vi "sub UI set title.vi"(8 "error in (no error)":errorcluster, 10 "title":T1, 11 "IDE simple in":refnum<class "LF2R IDE.lvclass">) -> (0 "error out":errorcluster, 3 "IDE simple out":refnum<class "LF2R IDE.lvclass">)   [LabVIEW 2018, in "LF2R IDE.lvlib" / "LF2R IDE.lvclass"]
uses:
  LF2R IDE.lvclass
  Frame Analizer/frame title.ctl
  LF2R IDE.lvclass/LF2R IDE.ctl
  Frame Analizer/Data Parser.lvclass
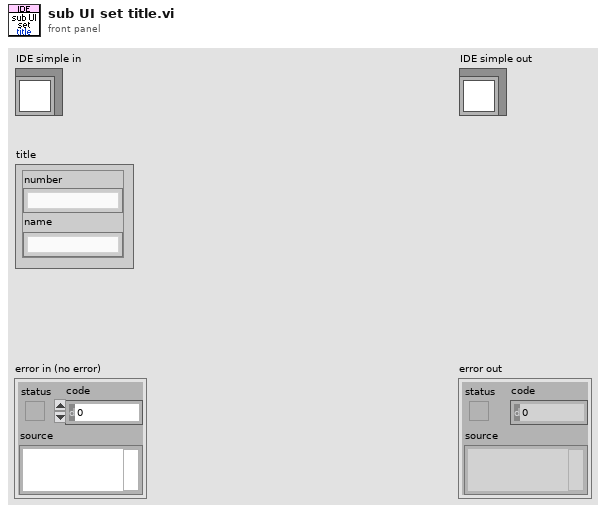
[diagram p1: front panel]
types:
  T1 = typedef "Data Parser.lvclass/frame title.ctl" = cluster{"number":string, "name":string}
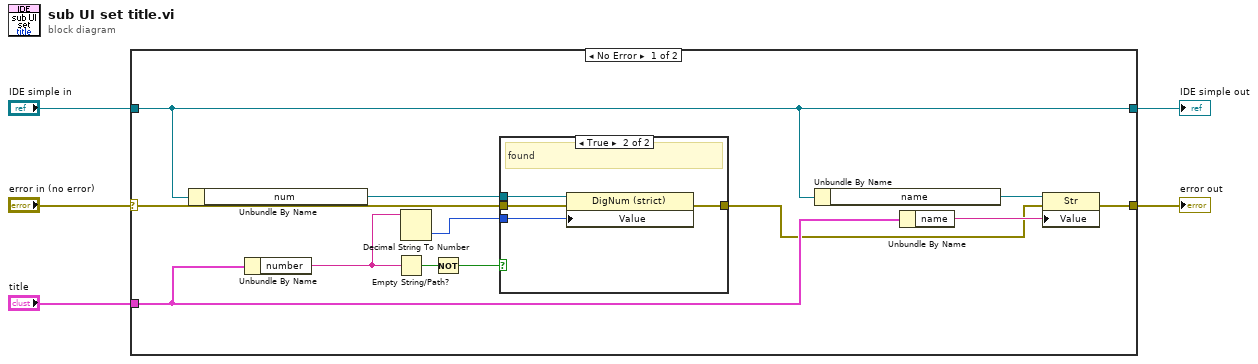
[diagram p0: block diagram]
diagram:
  n1 = case shown="No Error" "error in (no error)" {
    selector: "error in (no error)" -> [w7 w24]
    tunnel: [w15 w24] -> w4
    tunnel: [w14 w23] -> w2
    tunnel: "IDE simple in" -> [w14 w23]
    tunnel: "title" -> [w13 _]
    frame No Error {
      n2 = Unbundle By Name(w14) -> ("num"=w10:refnum<vi>)
      n3 = Unbundle By Name(w13) -> ("number"=w11:string)
      n4 = Empty String/Path?(string/path=w11) -> (empty?=w12:bool)
      n5 = Decimal String To Number(string=w11) -> (number=w8:i32)  [unwired: 2 in, 1 out]
      n6 = Not(x=w12) -> (.not. x?=w9:bool)
      n7 = case shown="True" w9 {
        tunnel: w10 -> [_ w22]
        tunnel: w8 -> [_ w21]
        tunnel: w7 -> [w18 w20]
        tunnel: [w18 w19] -> w6
        frame False {
          # "not found"
        }
        frame True {
          # "found"
          n8 = property class="DigNum (strict)"(reference=w22, error in=w20, "Value"=w21) -> (error out=w19:errorcluster)  [unwired: 1 out]
        }
      }
      n9 = Unbundle By Name(w14) -> ("name"=w17:refnum<vi>)
      n10 = Unbundle By Name(w13) -> ("name"=w16:string)
      n11 = property class="Str"(reference=w17, error in=w6, "Value"=w16) -> (error out=w15:errorcluster)  [unwired: 1 out]
    }
    frame Error {
    }
  }
  "error out" <- w4
  "IDE simple out" <- w2
